vi "FULL SUBTRACTOR.vi"(2 "C":bool, 3 "B":bool, 4 "A":bool) -> (0 "BORROW":bool, 1 "DIFF":bool)   [LabVIEW 2011]
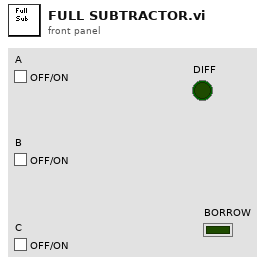
[diagram p1: front panel]
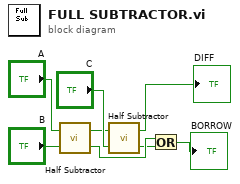
[diagram p0: block diagram]
diagram:
  n1 = call "Half Subtractor.vi"("B"="B", "A"="A") -> ("BORROW"=w5:bool, "DIFF"=w1:bool)
  n2 = call "Half Subtractor.vi"("B"="C", "A"=w1) -> ("BORROW"=w4:bool, "DIFF"=→"DIFF":bool)
  n3 = Or(x=w5, y=w4) -> (x .or. y?=→"BORROW":bool)
